vi "GUNSC_test.vi"() -> ()   [LabVIEW 2014]
uses:
  ctest/libmap.so
  Common/Clib/lib/libmem.so.20
  expglobal.vi
  flags.vi
panel:
  in  "writekey command":string
  in  "send unsc":bool
  in  "send geom":bool
  in  "Geometry command":string
  in  "new unscrambled image":path=path "/home/ArcVIEW/Modules/GUNSC/test/ctest/test"
  in  "multiple extensions":bool=TRUE
  in  "ReadModes":u16(ring) items=["4ch", ""]
  in  "FPA name":string="KIRMOS"
  in  "error in (no error)":errorcluster
  in  "naxis":i32
  in  "bitpix":i32
  in  "nrows":i32
  in  "ncols":i32
  in  "scramble image on disk":path=path "/home/ArcVIEW/Modules/GUNSC/test/ctest/scr.fits"
  in  "stop":bool
  in  "Pieces":u16=1 min=1
  in  "send":bool
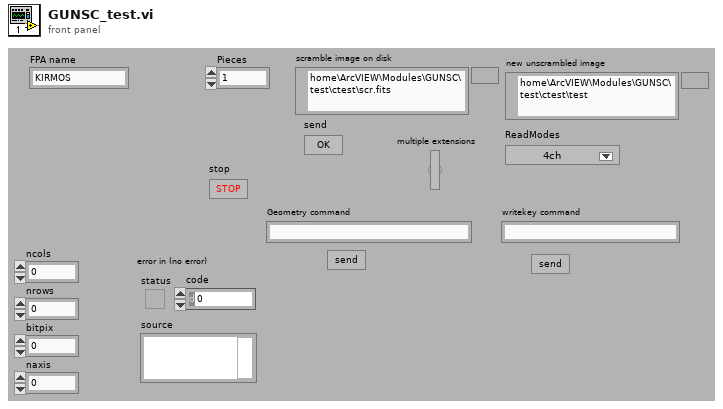
[diagram p1: front panel]
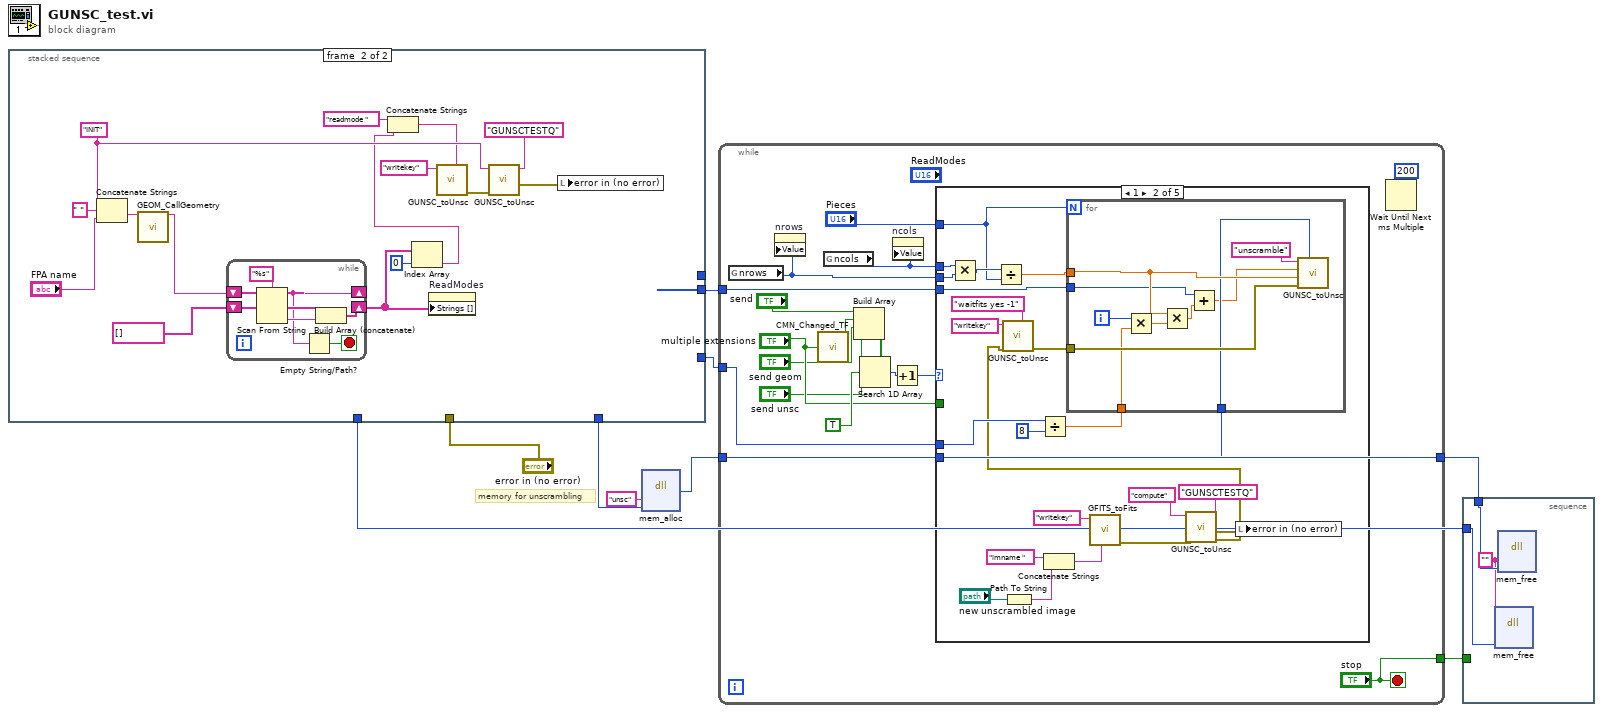
[diagram p0: block diagram]
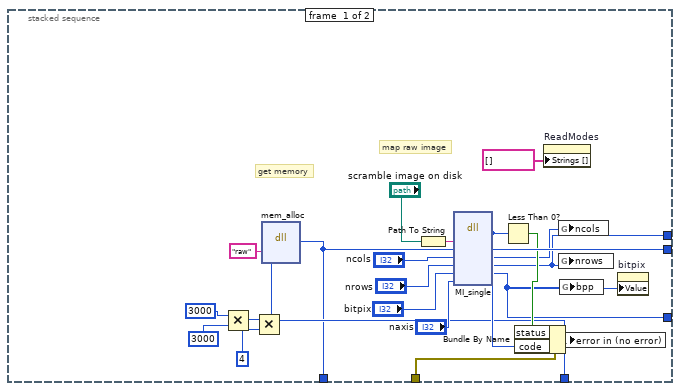
[diagram p2: hidden frame]
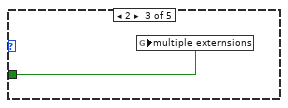
[diagram p4: hidden frame]
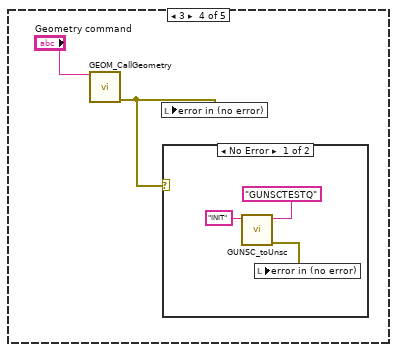
[diagram p5: hidden frame]
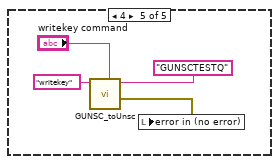
[diagram p7: hidden frame]
diagram:
  # "memory for unscrambling"
  n1 = stacked-sequence {
    tunnel: [w20 _] -> w9
    tunnel: "error in (no error)" -> [w17 _]
    tunnel: [w15 _] -> w6
    tunnel: [w12 _] -> _
    tunnel: [w11 _] -> w4
    tunnel: [w10 _] -> w1
    frame #0 {
      # "get memory"
      # "map raw image"
      n2 = Multiply(x=3000, y=3000) -> (x*y=w21:i32)
      n3 = Multiply(x=w21, y=4) -> (x*y=w15:i32)
      n4 = dll-call lib="home/sispi/Panview-1.13.0-64b/PAN/Modules/Common/Clib/lib/libmem.so.20" fn="mem_alloc"("name"="raw", "size"=w15) -> (w10:u32)  [unwired: 5 in, 2 out]
      n5 = Path To String(path="scramble image on disk") -> (string=w31:string)
      n6 = dll-call lib="uyq0/home/bonati/PAN/Modules/GUNSC/test/ctest/libmap.so" fn="MI_single"("filename"=w31, "map_addr"=w10, "ncols"="ncols", "nrows"="nrows", "bitpix"="bitpix", "naxis"="naxis") -> (w18:i32, "map_addr"=w20:u32, "ncols"=w13:i32, "nrows"=w12:i32, "bitpix"=w11:i32)  [unwired: 5 in, 2 out]
      n7 = Less Than 0?(x=w18) -> (x < 0?=w19:bool)
      n8 = Bundle By Name(cluster=w17, "status"=w19, "code"=w18) -> (w16:errorcluster)
      n9 = property on="ReadModes" class="Ring (strict)"("Strings []"=string[] []) -> ()  [unwired: 2 in, 2 out]
      n10 = global write "expglobal.vi" "ncols"(w13) -> ()
      n11 = global write "expglobal.vi" "nrows"(w12) -> ()
      n12 = global write "expglobal.vi" "bpp"(w11) -> ()
      n13 = local write "error in (no error)"(w16) -> ()
      n14 = property on="bitpix" class="DigNum (strict)"("Value"=w11) -> ()  [unwired: 2 in, 2 out]
    }
    frame #1 {
      w46 = "INIT" ("string")
      n15 = Concatenate Strings(w46, " " ("string"), "FPA name") -> (w44:string)
      n16 = call "GEOM_CallGeometry.vi"("Command"=w44) -> ("ImmedReplyString"=w35:string)  [unwired: 13 in, 1 out]
      n17 = while {
        shift-right: [w51] -> w33
        shift-left: string[] [] -> [w50]
        shift-right: [w47] -> _
        shift-left: w35 -> [w49]
        stop <- w48 stop-if-true
        n18 = Scan From String(format string="%s", input string=w49) -> (remaining string=w47:string, output 1=w52:string)  [unwired: 3 in, 2 out]
        n19 = Empty String/Path?(string/path=w47) -> (empty?=w48:bool)
        n20 = Build Array (concatenate)(w50, w52) -> (w51:string[])
      }
      n21 = Index Array(array=w33, index=0) -> (element=w38:string)
      n22 = Concatenate Strings("readmode " ("string"), w38) -> (w37:string)
      n23 = property on="ReadModes" class="Ring (strict)"("Strings []"=w33) -> ()  [unwired: 2 in, 2 out]
      n24 = call "GUNSC_toUnsc.vi"("key"=w37, "command"="writekey") -> ("error out"=w42:errorcluster)  [unwired: 8 in, 1 out]
      n25 = call "GUNSC_toUnsc.vi"("responseQ"="GUNSCTESTQ", "error in (no error)"=w42, "command"=w46) -> ("response"=w32:errorcluster)  [unwired: 7 in, 1 out]
      n26 = local write "error in (no error)"(w32) -> ()
    }
  }
  n27 = dll-call lib="home/sispi/Panview-1.13.0-64b/PAN/Modules/Common/Clib/lib/libmem.so.20" fn="mem_alloc"("name"="unsc", "size"=w6) -> (w5:u32)  [unwired: 5 in, 2 out]
  n28 = while {
    tunnel: w9 -> [w63]
    tunnel: w5 -> [w58]
    tunnel: w4 -> [w62]
    tunnel: ["stop"] -> w3
    tunnel: [w58] -> w2
    stop <- "stop" stop-if-true
    n29 = global read "expglobal.vi" "nrows"() -> (w55:u32)
    n30 = property on="nrows" class="DigNum (strict)"("Value"=w55) -> ()  [unwired: 2 in, 2 out]
    n31 = call "CMN_Changed_TF.vi"("value"="multiple extensions") -> ("changed?"=w61:bool)  [unwired: 4 in]
    n32 = global read "expglobal.vi" "ncols"() -> (w56:u32)
    n33 = Build Array("send", w61, "send geom", "send unsc") -> (w68:bool[])
    n34 = Search 1D Array(1D array=w68, element=TRUE) -> (index of element=w66:i32)  [unwired: 1 in]
    n35 = Increment(x=w66) -> (x+1=w65:i32)
    n36 = property on="ncols" class="DigNum (strict)"("Value"=w56) -> ()  [unwired: 2 in, 2 out]
    n37 = case shown="1" w65 {
      tunnel: "Pieces" -> [_ w89 _ _ _]
      tunnel: w58 -> [_ w93 _ _ _]
      tunnel: w63 -> [_ w84 _ _ _]
      tunnel: w56 -> [_ w92 _ _ _]
      tunnel: w55 -> [_ w91 _ _ _]
      tunnel: w62 -> [_ w83 _ _ _]
      tunnel: "multiple extensions" -> [_ _ w104 _ _]
      frame 0, Default {
      }
      frame 1 {
        n38 = Multiply(x=w92, y=w91) -> (x*y=w90:u32)
        n39 = Divide(x=w90, y=w89) -> (x/y=w88:dbl)
        n40 = Path To String(path="new unscrambled image") -> (string=w73:string)
        n41 = Divide(x=w83, y=8) -> (x/y=w81:dbl)
        n42 = Concatenate Strings("imname " ("string"), w73) -> (w72:string)
        n43 = call "GFITS_toFits.vi"("key"=w72, "command"="writekey") -> ("error out"=w77:errorcluster)  [unwired: 8 in, 1 out]
        n44 = call "GUNSC_toUnsc.vi"("responseQ"="GUNSCTESTQ", "error in (no error)"=w77, "command"="compute") -> ("error out"=w71:errorcluster, "response"=w78:errorcluster)  [unwired: 7 in]
        n45 = call "GUNSC_toUnsc.vi"("key"="waitfits yes -1", "error in (no error)"=w71, "command"="writekey") -> ("error out"=w85:errorcluster)  [unwired: 7 in, 1 out]
        n46 = for {
          N: w89 -> [_]
          tunnel: w93 -> [w95]
          tunnel: w88 -> [w98]
          tunnel: w85 -> [w102]
          tunnel: w84 -> [w96]
          tunnel: w81 -> [w100]
          i -> [w101]
          n47 = Multiply(x=w101, y=w100) -> (x*y=w99:dbl)
          n48 = Multiply(x=w98, y=w99) -> (x*y=w97:dbl)
          n49 = Add(x=w96, y=w97) -> (x+y=w94:dbl)
          n50 = call "GUNSC_toUnsc.vi"("location 2"=w95, "error in (no error)"=w102, "ele Read"=w98, "location"=w94, "command"="unscramble") -> ()  [unwired: 5 in, 2 out]
        }
        n51 = local write "error in (no error)"(w78) -> ()
      }
      frame 2 {
        n52 = global write "flags.vi" "multiple externsions"(w104) -> ()
      }
      frame 3 {
        n53 = call "GEOM_CallGeometry.vi"("Command"="Geometry command") -> ("error out"=w105:errorcluster)  [unwired: 13 in, 1 out]
        n54 = local write "error in (no error)"(w105) -> ()
        n55 = case shown="No Error" w105 {
          frame No Error {
            n56 = call "GUNSC_toUnsc.vi"("responseQ"="GUNSCTESTQ", "command"="INIT") -> ("error out"=w107:errorcluster)  [unwired: 8 in, 1 out]
            n57 = local write "error in (no error)"(w107) -> ()
          }
          frame Error {
          }
        }
      }
      frame 4 {
        n58 = call "GUNSC_toUnsc.vi"("responseQ"="GUNSCTESTQ", "key"="writekey command", "command"="writekey") -> ("response"=w112:errorcluster)  [unwired: 7 in, 1 out]
        n59 = local write "error in (no error)"(w112) -> ()
      }
    }
    n60 = Wait Until Next ms Multiple(millisecond multiple=u32 200) -> ()  [unwired: 1 out]
  }
  n61 = stacked-sequence {
    tunnel: w3 -> [_]
    tunnel: w2 -> [w116]
    tunnel: w1 -> [w115]
    frame #0 {
      w114 = "" ("name")
      n62 = dll-call lib="home/sispi/Panview-1.13.0-64b/PAN/Modules/Common/Clib/lib/libmem.so.20" fn="mem_free"("name"=w114, "location"=w115) -> ()  [unwired: 6 in, 2 out]
      n63 = dll-call lib="home/sispi/Panview-1.13.0-64b/PAN/Modules/Common/Clib/lib/libmem.so.20" fn="mem_free"("name"=w114, "location"=w116) -> ()  [unwired: 6 in, 2 out]
    }
  }
